vi "PCO_GetDSNUAdjustMode.vi"(0 "ph":u64, 11 "error in (no error)":errorcluster {"code" format="%x"}) -> (4 "ph out":u64, 6 "ErrorMessage":i32 format="%x", 8 "wDSNUAdjustMode":u16(ring) items=["No DSNU Correction", "Auto DSNU Correction", "Manual DSNU Correction"], 15 "error out":errorcluster {"code" format="%x"})   [LabVIEW 2019, in "SDK.lvlib" / "ImageSensor.lvlib"]
doc: "Returns the current state of the DSNU correction"
uses:
  ImageSensor.lvlib
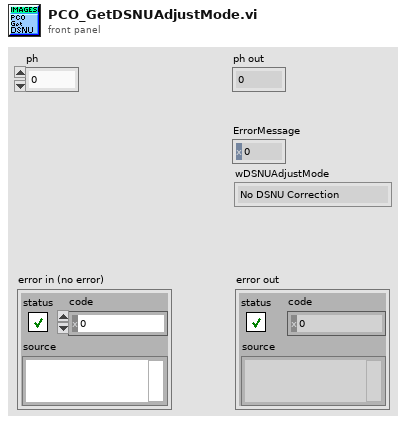
[diagram p1: front panel]
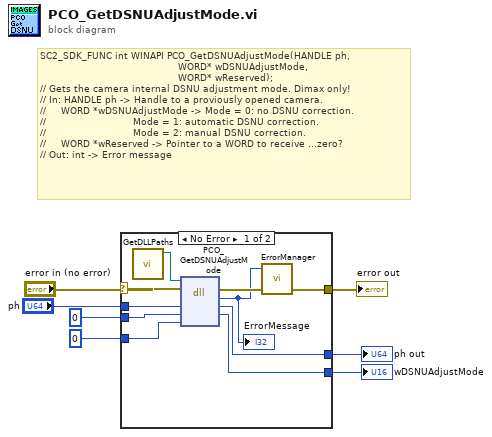
[diagram p0: block diagram]
diagram:
  # "SC2_SDK_FUNC int WINAPI PCO_GetDSNUAdjustMode(HANDLE ph,\n                                              WORD* wDSNUAdjustMode,\n                                              WORD* wReserved);\n// Gets the camera internal DSNU adjustment mode. Dimax only!\n// In: HANDLE ph -> Handle to a proviously opened camera.\n//     WORD *wDSNUAdjustMode -> Mode = 0: no DSNU correction.\n//                             Mode = 1: automatic DSNU correction.\n//                             Mode = 2: manual DSNU correction.\n//     WORD *wReserved -> Pointer to a WORD to receive ...zero?\n// Out: int -> Error message"
  n1 = case shown="No Error" "error in (no error)" {
    selector: "error in (no error)" -> [w10 w20]
    tunnel: "ph" -> [w17 w19]
    tunnel: [w16 w19] -> w6
    tunnel: u16 0 ("wNoiseFilterMode") -> [w15 w18]
    tunnel: [w14 w18] -> w4
    tunnel: [w12 w20] -> w3
    tunnel: u16 0 ("wReserved") -> [w8 _]
    frame No Error {
      n2 = call "GetDLLPaths.vi"() -> ("SC2_Cam_Path"=w9:path)  [unwired: 8 in, 3 out]
      n3 = dll-call lib="?" fn="PCO_GetDSNUAdjustMode"(path in=w9, error in=w10, "ph"=w17, "wDSNUAdjustMode"=w15, "wReserved"=w8) -> (error out=w13:errorcluster, "return type"=w11:i32, "ph"=w16:u64, "wDSNUAdjustMode"=w14:u16)  [unwired: 2 in, 1 out]
      "ErrorMessage" <- w11
      n4 = call "ErrorManager.vi"("error in (no error)"=w13, "error code"=w11) -> ("error out"=w12:errorcluster)  [unwired: 2 in, 1 out]
    }
    frame Error {
    }
  }
  "ph out" <- w6
  "wDSNUAdjustMode" <- w4
  "error out" <- w3
